vi "Array_Functions.vi"() -> ()   [LabVIEW 2024]
panel:
  out "descending array":dbl[](array[numeric])
  out "size":i32
  out "max value":dbl
  out "max index(es)":i32
  out "min value":dbl
  out "min index(es)":i32
  out "sorted array":dbl[](array[numeric])
  out "outputArray":dbl[](array[numeric])
  in  "Numeric":dbl
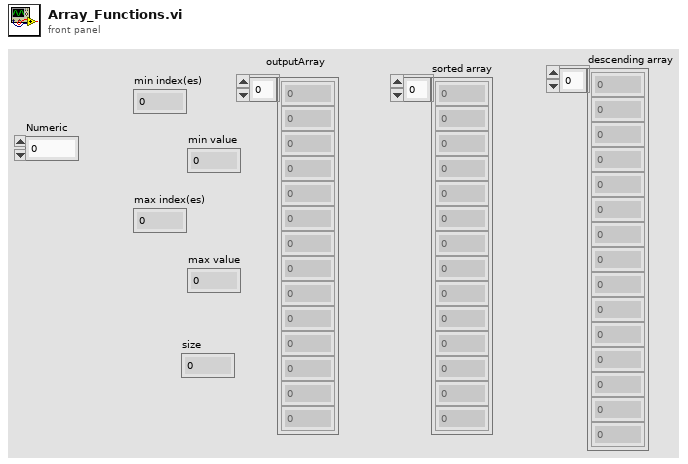
[diagram p1: front panel]
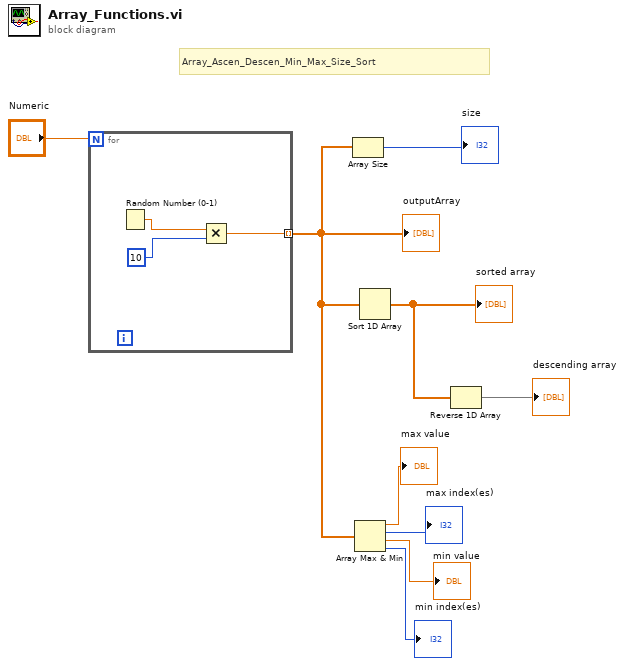
[diagram p0: block diagram]
diagram:
  # "Array_Ascen_Descen_Min_Max_Size_Sort"
  n1 = for {
    N: "Numeric" -> [_]
    tunnel: [w10] -> w2 mode=indexing
    n2 = Random Number (0-1)() -> (number: 0 to 1=w12:dbl)
    n3 = Multiply(x=w12, y=10) -> (x*y=w10:dbl)
  }
  "outputArray" <- w2
  n4 = Array Size(array=w2) -> (size(s)=→"size":i32)
  n5 = Array Max & Min(array=w2) -> (max value=→"max value":dbl, max index (indices)=→"max index(es)":i32, min value=→"min value":dbl, min index (indices)=→"min index(es)":i32)
  n6 = Sort 1D Array(array=w2) -> (sorted array=w1:dbl[])
  "sorted array" <- w1
  n7 = Reverse 1D Array(array=w1) -> (reversed array=→"descending array":dbl[])
